vi "fit_fix height and width.vi"() -> ()   [LabVIEW 2016] (continued)
-3.5199999999999996, -3.4799999999999995, -3.4399999999999995, -3.3999999999999995, -3.3600000000000003, -3.3200000000000003, -3.2800000000000002, -3.24, -3.2, -3.16, -3.12, -3.08, -3.04], []}, {[-9.0, -8.96, -8.92, -8.88, -8.84, -8.8, -8.76, -8.72, -8.68, -8.64, -8.6, -8.56, -8.52, -8.48, -8.44, -8.4, -8.36, -8.32, -8.28, -8.24, -8.2, -8.16, -8.12, -8.08, -8.04, -8.0, -7.96, -7.92, -7.88, -7.84, -7.8, -7.76, -7.72, -7.68, -7.64, -7.6, -7.5600000000000005, -7.52, -7.48, -7.4399999999999995, -7.4, -7.359999999999999, -7.32, -7.28, -7.24, -7.2, -7.16, -7.12, -7.08, -7.04, -7.0, -6.96, -6.92, -6.88, -6.84, -6.8, -6.76, -6.72, -6.68, -6.640000000000001, -6.6, -6.5600000000000005, -6.52, -6.48, -6.4399999999999995, -6.4, -6.359999999999999, -6.32, -6.279999999999999, -6.24, -6.199999999999999, -6.16, -6.12, -6.08, -6.04, -6.0, -5.96, -5.92, -5.88, -5.84, -5.8, -5.76, -5.72, -5.68, -5.640000000000001, -5.6, -5.5600000000000005, -5.52, -5.48, -5.4399999999999995, -5.4, -5.359999999999999, -5.32, -5.279999999999999, -5.24, -5.199999999999999, -5.16, -5.12, -5.08, -5.04, -5.0, -4.96, -4.92, -4.88, -4.84, -4.8, -4.76, -4.72, -4.68, -4.64, -4.6, -4.56, -4.52, -4.4799999999999995, -4.4399999999999995, -4.3999999999999995, -4.36, -4.32, -4.28, -4.24, -4.2, -4.16, -4.12, -4.08, -4.04, -4.0, -3.96, -3.92, -3.88, -3.84, -3.8, -3.76, -3.7199999999999998, -3.6799999999999997, -3.6399999999999997, -3.5999999999999996, -3.5599999999999996, -3.5199999999999996, -3.4799999999999995, -3.4399999999999995, -3.3999999999999995, -3.3600000000000003, -3.3200000000000003, -3.2800000000000002, -3.24, -3.2, -3.16, -3.12, -3.08, -3.04], []}, {[-9.0, -8.96, -8.92, -8.88, -8.84, -8.8, -8.76, -8.72, -8.68, -8.64, -8.6, -8.56, -8.52, -8.48, -8.44, -8.4, -8.36, -8.32, -8.28, -8.24, -8.2, -8.16, -8.12, -8.08, -8.04, -8.0, -7.96, -7.92, -7.88, -7.84, -7.8, -7.76, -7.72, -7.68, -7.64, -7.6, -7.5600000000000005, -7.52, -7.48, -7.4399999999999995, -7.4, -7.359999999999999, -7.32, -7.28, -7.24, -7.2, -7.16, -7.12, -7.08, -7.04, -7.0, -6.96, -6.92, -6.88, -6.84, -6.8, -6.76, -6.72, -6.68, -6.640000000000001, -6.6, -6.5600000000000005, -6.52, -6.48, -6.4399999999999995, -6.4, -6.359999999999999, -6.32, -6.279999999999999, -6.24, -6.199999999999999, -6.16, -6.12, -6.08, -6.04, -6.0, -5.96, -5.92, -5.88, -5.84, -5.8, -5.76, -5.72, -5.68, -5.640000000000001, -5.6, -5.5600000000000005, -5.52, -5.48, -5.4399999999999995, -5.4, -5.359999999999999, -5.32, -5.279999999999999, -5.24, -5.199999999999999, -5.16, -5.12, -5.08, -5.04, -5.0, -4.96, -4.92, -4.88, -4.84, -4.8, -4.76, -4.72, -4.68, -4.64, -4.6, -4.56, -4.52, -4.4799999999999995, -4.4399999999999995, -4.3999999999999995, -4.36, -4.32, -4.28, -4.24, -4.2, -4.16, -4.12, -4.08, -4.04, -4.0, -3.96, -3.92, -3.88, -3.84, -3.8, -3.76, -3.7199999999999998, -3.6799999999999997, -3.6399999999999997, -3.5999999999999996, -3.5599999999999996, -3.5199999999999996, -3.4799999999999995, -3.4399999999999995, -3.3999999999999995, -3.3600000000000003, -3.3200000000000003, -3.2800000000000002, -3.24, -3.2, -3.16, -3.12, -3.08, -3.04], []}, {[-9.0, -8.96, -8.92, -8.88, -8.84, -8.8, -8.76, -8.72, -8.68, -8.64, -8.6, -8.56, -8.52, -8.48, -8.44, -8.4, -8.36, -8.32, -8.28, -8.24, -8.2, -8.16, -8.12, -8.08, -8.04, -8.0, -7.96, -7.92, -7.88, -7.84, -7.8, -7.76, -7.72, -7.68, -7.64, -7.6, -7.5600000000000005, -7.52, -7.48, -7.4399999999999995, -7.4, -7.359999999999999, -7.32, -7.28, -7.24, -7.2, -7.16, -7.12, -7.08, -7.04, -7.0, -6.96, -6.92, -6.88, -6.84, -6.8, -6.76, -6.72, -6.68, -6.640000000000001, -6.6, -6.5600000000000005, -6.52, -6.48, -6.4399999999999995, -6.4, -6.359999999999999, -6.32, -6.279999999999999, -6.24, -6.199999999999999, -6.16, -6.12, -6.08, -6.04, -6.0, -5.96, -5.92, -5.88, -5.84, -5.8, -5.76, -5.72, -5.68, -5.640000000000001, -5.6, -5.5600000000000005, -5.52, -5.48, -5.4399999999999995, -5.4, -5.359999999999999, -5.32, -5.279999999999999, -5.24, -5.199999999999999, -5.16, -5.12, -5.08, -5.04, -5.0, -4.96, -4.92, -4.88, -4.84, -4.8, -4.76, -4.72, -4.68, -4.64, -4.6, -4.56, -4.52, -4.4799999999999995, -4.4399999999999995, -4.3999999999999995, -4.36, -4.32, -4.28, -4.24, -4.2, -4.16, -4.12, -4.08, -4.04, -4.0, -3.96, -3.92, -3.88, -3.84, -3.8, -3.76, -3.7199999999999998, -3.6799999999999997, -3.6399999999999997, -3.5999999999999996, -3.5599999999999996, -3.5199999999999996, -3.4799999999999995, -3.4399999999999995, -3.3999999999999995, -3.3600000000000003, -3.3200000000000003, -3.2800000000000002, -3.24, -3.2, -3.16, -3.12, -3.08, -3.04], []}, {[-9.0, -8.96, -8.92, -8.88, -8.84, -8.8, -8.76, -8.72, -8.68, -8.64, -8.6, -8.56, -8.52, -8.48, -8.44, -8.4, -8.36, -8.32, -8.28, -8.24, -8.2, -8.16, -8.12, -8.08, -8.04, -8.0, -7.96, -7.92, -7.88, -7.84, -7.8, -7.76, -7.72, -7.68, -7.64, -7.6, -7.5600000000000005, -7.52, -7.48, -7.4399999999999995, -7.4, -7.359999999999999, -7.32, -7.28, -7.24, -7.2, -7.16, -7.12, -7.08, -7.04, -7.0, -6.96, -6.92, -6.88, -6.84, -6.8, -6.76, -6.72, -6.68, -6.640000000000001, -6.6, -6.5600000000000005, -6.52, -6.48, -6.4399999999999995, -6.4, -6.359999999999999, -6.32, -6.279999999999999, -6.24, -6.199999999999999, -6.16, -6.12, -6.08, -6.04, -6.0, -5.96, -5.92, -5.88, -5.84, -5.8, -5.76, -5.72, -5.68, -5.640000000000001, -5.6, -5.5600000000000005, -5.52, -5.48, -5.4399999999999995, -5.4, -5.359999999999999, -5.32, -5.279999999999999, -5.24, -5.199999999999999, -5.16, -5.12, -5.08, -5.04, -5.0, -4.96, -4.92, -4.88, -4.84, -4.8, -4.76, -4.72, -4.68, -4.64, -4.6, -4.56, -4.52, -4.4799999999999995, -4.4399999999999995, -4.3999999999999995, -4.36, -4.32, -4.28, -4.24, -4.2, -4.16, -4.12, -4.08, -4.04, -4.0, -3.96, -3.92, -3.88, -3.84, -3.8, -3.76, -3.7199999999999998, -3.6799999999999997, -3.6399999999999997, -3.5999999999999996, -3.5599999999999996, -3.5199999999999996, -3.4799999999999995, -3.4399999999999995, -3.3999999999999995, -3.3600000000000003, -3.3200000000000003, -3.2800000000000002, -3.24, -3.2, -3.16, -3.12, -3.08, -3.04], []}, {[-9.0, -8.96, -8.92, -8.88, -8.84, -8.8, -8.76, -8.72, -8.68, -8.64, -8.6, -8.56, -8.52, -8.48, -8.44, -8.4, -8.36, -8.32, -8.28, -8.24, -8.2, -8.16, -8.12, -8.08, -8.04, -8.0, -7.96, -7.92, -7.88, -7.84, -7.8, -7.76, -7.72, -7.68, -7.64, -7.6, -7.5600000000000005, -7.52, -7.48, -7.4399999999999995, -7.4, -7.359999999999999, -7.32, -7.28, -7.24, -7.2, -7.16, -7.12, -7.08, -7.04, -7.0, -6.96, -6.92, -6.88, -6.84, -6.8, -6.76, -6.72, -6.68, -6.640000000000001, -6.6, -6.5600000000000005, -6.52, -6.48, -6.4399999999999995, -6.4, -6.359999999999999, -6.32, -6.279999999999999, -6.24, -6.199999999999999, -6.16, -6.12, -6.08, -6.04, -6.0, -5.96, -5.92, -5.88, -5.84, -5.8, -5.76, -5.72, -5.68, -5.640000000000001, -5.6, -5.5600000000000005, -5.52, -5.48, -5.4399999999999995, -5.4, -5.359999999999999, -5.32, -5.279999999999999, -5.24, -5.199999999999999, -5.16, -5.12, -5.08, -5.04, -5.0, -4.96, -4.92, -4.88, -4.84, -4.8, -4.76, -4.72, -4.68, -4.64, -4.6, -4.56, -4.52, -4.4799999999999995, -4.4399999999999995, -4.3999999999999995, -4.36, -4.32, -4.28, -4.24, -4.2, -4.16, -4.12, -4.08, -4.04, -4.0, -3.96, -3.92, -3.88, -3.84, -3.8, -3.76, -3.7199999999999998, -3.6799999999999997, -3.6399999999999997, -3.5999999999999996, -3.5599999999999996, -3.5199999999999996, -3.4799999999999995, -3.4399999999999995, -3.3999999999999995, -3.3600000000000003, -3.3200000000000003, -3.2800000000000002, -3.24, -3.2, -3.16, -3.12, -3.08, -3.04], []}, {[-9.0, -8.96, -8.92, -8.88, -8.84, -8.8, -8.76, -8.72, -8.68, -8.64, -8.6, -8.56, -8.52, -8.48, -8.44, -8.4, -8.36, -8.32, -8.28, -8.24, -8.2, -8.16, -8.12, -8.08, -8.04, -8.0, -7.96, -7.92, -7.88, -7.84, -7.8, -7.76, -7.72, -7.68, -7.64, -7.6, -7.5600000000000005, -7.52, -7.48, -7.4399999999999995, -7.4, -7.359999999999999, -7.32, -7.28, -7.24, -7.2, -7.16, -7.12, -7.08, -7.04, -7.0, -6.96, -6.92, -6.88, -6.84, -6.8, -6.76, -6.72, -6.68, -6.640000000000001, -6.6, -6.5600000000000005, -6.52, -6.48, -6.4399999999999995, -6.4, -6.359999999999999, -6.32, -6.279999999999999, -6.24, -6.199999999999999, -6.16, -6.12, -6.08, -6.04, -6.0, -5.96, -5.92, -5.88, -5.84, -5.8, -5.76, -5.72, -5.68, -5.640000000000001, -5.6, -5.5600000000000005, -5.52, -5.48, -5.4399999999999995, -5.4, -5.359999999999999, -5.32, -5.279999999999999, -5.24, -5.199999999999999, -5.16, -5.12, -5.08, -5.04, -5.0, -4.96, -4.92, -4.88, -4.84, -4.8, -4.76, -4.72, -4.68, -4.64, -4.6, -4.56, -4.52, -4.4799999999999995, -4.4399999999999995, -4.3999999999999995, -4.36, -4.32, -4.28, -4.24, -4.2, -4.16, -4.12, -4.08, -4.04, -4.0, -3.96, -3.92, -3.88, -3.84, -3.8, -3.76, -3.7199999999999998, -3.6799999999999997, -3.6399999999999997, -3.5999999999999996, -3.5599999999999996, -3.5199999999999996, -3.4799999999999995, -3.4399999999999995, -3.3999999999999995, -3.3600000000000003, -3.3200000000000003, -3.2800000000000002, -3.24, -3.2, -3.16, -3.12, -3.08, -3.04], []}, {[-9.0, -8.96, -8.92, -8.88, -8.84, -8.8, -8.76, -8.72, -8.68, -8.64, -8.6, -8.56, -8.52, -8.48, -8.44, -8.4, -8.36, -8.32, -8.28, -8.24, -8.2, -8.16, -8.12, -8.08, -8.04, -8.0, -7.96, -7.92, -7.88, -7.84, -7.8, -7.76, -7.72, -7.68, -7.64, -7.6, -7.5600000000000005, -7.52, -7.48, -7.4399999999999995, -7.4, -7.359999999999999, -7.32, -7.28, -7.24, -7.2, -7.16, -7.12, -7.08, -7.04, -7.0, -6.96, -6.92, -6.88, -6.84, -6.8, -6.76, -6.72, -6.68, -6.640000000000001, -6.6, -6.5600000000000005, -6.52, -6.48, -6.4399999999999995, -6.4, -6.359999999999999, -6.32, -6.279999999999999, -6.24, -6.199999999999999, -6.16, -6.12, -6.08, -6.04, -6.0, -5.96, -5.92, -5.88, -5.84, -5.8, -5.76, -5.72, -5.68, -5.640000000000001, -5.6, -5.5600000000000005, -5.52, -5.48, -5.4399999999999995, -5.4, -5.359999999999999, -5.32, -5.279999999999999, -5.24, -5.199999999999999, -5.16, -5.12, -5.08, -5.04, -5.0, -4.96, -4.92, -4.88, -4.84, -4.8, -4.76, -4.72, -4.68, -4.64, -4.6, -4.56, -4.52, -4.4799999999999995, -4.4399999999999995, -4.3999999999999995, -4.36, -4.32, -4.28, -4.24, -4.2, -4.16, -4.12, -4.08, -4.04, -4.0, -3.96, -3.92, -3.88, -3.84, -3.8, -3.76, -3.7199999999999998, -3.6799999999999997, -3.6399999999999997, -3.5999999999999996, -3.5599999999999996, -3.5199999999999996, -3.4799999999999995, -3.4399999999999995, -3.3999999999999995, -3.3600000000000003, -3.3200000000000003, -3.2800000000000002, -3.24, -3.2, -3.16, -3.12, -3.08, -3.04], []}, {[-9.0, -8.96, -8.92, -8.88, -8.84, -8.8, -8.76, -8.72, -8.68, -8.64, -8.6, -8.56, -8.52, -8.48, -8.44, -8.4, -8.36, -8.32, -8.28, -8.24, -8.2, -8.16, -8.12, -8.08, -8.04, -8.0, -7.96, -7.92, -7.88, -7.84, -7.8, -7.76, -7.72, -7.68, -7.64, -7.6, -7.5600000000000005, -7.52, -7.48, -7.4399999999999995, -7.4, -7.359999999999999, -7.32, -7.28, -7.24, -7.2, -7.16, -7.12, -7.08, -7.04, -7.0, -6.96, -6.92, -6.88, -6.84, -6.8, -6.76, -6.72, -6.68, -6.640000000000001, -6.6, -6.5600000000000005, -6.52, -6.48, -6.4399999999999995, -6.4, -6.359999999999999, -6.32, -6.279999999999999, -6.24, -6.199999999999999, -6.16, -6.12, -6.08, -6.04, -6.0, -5.96, -5.92, -5.88, -5.84, -5.8, -5.76, -5.72, -5.68, -5.640000000000001, -5.6, -5.5600000000000005, -5.52, -5.48, -5.4399999999999995, -5.4, -5.359999999999999, -5.32, -5.279999999999999, -5.24, -5.199999999999999, -5.16, -5.12, -5.08, -5.04, -5.0, -4.96, -4.92, -4.88, -4.84, -4.8, -4.76, -4.72, -4.68, -4.64, -4.6, -4.56, -4.52, -4.4799999999999995, -4.4399999999999995, -4.3999999999999995, -4.36, -4.32, -4.28, -4.24, -4.2, -4.16, -4.12, -4.08, -4.04, -4.0, -3.96, -3.92, -3.88, -3.84, -3.8, -3.76, -3.7199999999999998, -3.6799999999999997, -3.6399999999999997, -3.5999999999999996, -3.5599999999999996, -3.5199999999999996, -3.4799999999999995, -3.4399999999999995, -3.3999999999999995, -3.3600000000000003, -3.3200000000000003, -3.2800000000000002, -3.24, -3.2, -3.16, -3.12, -3.08, -3.04], []}, {[-9.0, -8.96, -8.92, -8.88, -8.84, -8.8, -8.76, -8.72, -8.68, -8.64, -8.6, -8.56, -8.52, -8.48, -8.44, -8.4, -8.36, -8.32, -8.28, -8.24, -8.2, -8.16, -8.12, -8.08, -8.04, -8.0, -7.96, -7.92, -7.88, -7.84, -7.8, -7.76, -7.72, -7.68, -7.64, -7.6, -7.5600000000000005, -7.52, -7.48, -7.4399999999999995, -7.4, -7.359999999999999, -7.32, -7.28, -7.24, -7.2, -7.16, -7.12, -7.08, -7.04, -7.0, -6.96, -6.92, -6.88, -6.84, -6.8, -6.76, -6.72, -6.68, -6.640000000000001, -6.6, -6.5600000000000005, -6.52, -6.48, -6.4399999999999995, -6.4, -6.359999999999999, -6.32, -6.279999999999999, -6.24, -6.199999999999999, -6.16, -6.12, -6.08, -6.04, -6.0, -5.96, -5.92, -5.88, -5.84, -5.8, -5.76, -5.72, -5.68, -5.640000000000001, -5.6, -5.5600000000000005, -5.52, -5.48, -5.4399999999999995, -5.4, -5.359999999999999, -5.32, -5.279999999999999, -5.24, -5.199999999999999, -5.16, -5.12, -5.08, -5.04, -5.0, -4.96, -4.92, -4.88, -4.84, -4.8, -4.76, -4.72, -4.68, -4.64, -4.6, -4.56, -4.52, -4.4799999999999995, -4.4399999999999995, -4.3999999999999995, -4.36, -4.32, -4.28, -4.24, -4.2, -4.16, -4.12, -4.08, -4.04, -4.0, -3.96, -3.92, -3.88, -3.84, -3.8, -3.76, -3.7199999999999998, -3.6799999999999997, -3.6399999999999997, -3.5999999999999996, -3.5599999999999996, -3.5199999999999996, -3.4799999999999995, -3.4399999999999995, -3.3999999999999995, -3.3600000000000003, -3.3200000000000003, -3.2800000000000002, -3.24, -3.2, -3.16, -3.12, -3.08, -3.04], []}, {[-9.0, -8.96, -8.92, -8.88, -8.84, -8.8, -8.76, -8.72, -8.68, -8.64, -8.6, -8.56, -8.52, -8.48, -8.44, -8.4, -8.36, -8.32, -8.28, -8.24, -8.2, -8.16, -8.12, -8.08, -8.04, -8.0, -7.96, -7.92, -7.88, -7.84, -7.8, -7.76, -7.72, -7.68, -7.64, -7.6, -7.5600000000000005, -7.52, -7.48, -7.4399999999999995, -7.4, -7.359999999999999, -7.32, -7.28, -7.24, -7.2, -7.16, -7.12, -7.08, -7.04, -7.0, -6.96, -6.92, -6.88, -6.84, -6.8, -6.76, -6.72, -6.68, -6.640000000000001, -6.6, -6.5600000000000005, -6.52, -6.48, -6.4399999999999995, -6.4, -6.359999999999999, -6.32, -6.279999999999999, -6.24, -6.199999999999999, -6.16, -6.12, -6.08, -6.04, -6.0, -5.96, -5.92, -5.88, -5.84, -5.8, -5.76, -5.72, -5.68, -5.640000000000001, -5.6, -5.5600000000000005, -5.52, -5.48, -5.4399999999999995, -5.4, -5.359999999999999, -5.32, -5.279999999999999, -5.24, -5.199999999999999, -5.16, -5.12, -5.08, -5.04, -5.0, -4.96, -4.92, -4.88, -4.84, -4.8, -4.76, -4.72, -4.68, -4.64, -4.6, -4.56, -4.52, -4.4799999999999995, -4.4399999999999995, -4.3999999999999995, -4.36, -4.32, -4.28, -4.24, -4.2, -4.16, -4.12, -4.08, -4.04, -4.0, -3.96, -3.92, -3.88, -3.84, -3.8, -3.76, -3.7199999999999998, -3.6799999999999997, -3.6399999999999997, -3.5999999999999996, -3.5599999999999996, -3.5199999999999996, -3.4799999999999995, -3.4399999999999995, -3.3999999999999995, -3.3600000000000003, -3.3200000000000003, -3.2800000000000002, -3.24, -3.2, -3.16, -3.12, -3.08, -3.04], []}, {[-9.0, -8.96, -8.92, -8.88, -8.84, -8.8, -8.76, -8.72, -8.68, -8.64, -8.6, -8.56, -8.52, -8.48, -8.44, -8.4, -8.36, -8.32, -8.28, -8.24, -8.2, -8.16, -8.12, -8.08, -8.04, -8.0, -7.96, -7.92, -7.88, -7.84, -7.8, -7.76, -7.72, -7.68, -7.64, -7.6, -7.5600000000000005, -7.52, -7.48, -7.4399999999999995, -7.4, -7.359999999999999, -7.32, -7.28, -7.24, -7.2, -7.16, -7.12, -7.08, -7.04, -7.0, -6.96, -6.92, -6.88, -6.84, -6.8, -6.76, -6.72, -6.68, -6.640000000000001, -6.6, -6.5600000000000005, -6.52, -6.48, -6.4399999999999995, -6.4, -6.359999999999999, -6.32, -6.279999999999999, -6.24, -6.199999999999999, -6.16, -6.12, -6.08, -6.04, -6.0, -5.96, -5.92, -5.88, -5.84, -5.8, -5.76, -5.72, -5.68, -5.640000000000001, -5.6, -5.5600000000000005, -5.52, -5.48, -5.4399999999999995, -5.4, -5.359999999999999, -5.32, -5.279999999999999, -5.24, -5.199999999999999, -5.16, -5.12, -5.08, -5.04, -5.0, -4.96, -4.92, -4.88, -4.84, -4.8, -4.76, -4.72, -4.68, -4.64, -4.6, -4.56, -4.52, -4.4799999999999995, -4.4399999999999995, -4.3999999999999995, -4.36, -4.32, -4.28, -4.24, -4.2, -4.16, -4.12, -4.08, -4.04, -4.0, -3.96, -3.92, -3.88, -3.84, -3.8, -3.76, -3.7199999999999998, -3.6799999999999997, -3.6399999999999997, -3.5999999999999996, -3.5599999999999996, -3.5199999999999996, -3.4799999999999995, -3.4399999999999995, -3.3999999999999995, -3.3600000000000003, -3.3200000000000003, -3.2800000000000002, -3.24, -3.2, -3.16, -3.12, -3.08, -3.04], []}, {[-9.0, -8.96, -8.92, -8.88, -8.84, -8.8, -8.76, -8.72, -8.68, -8.64, -8.6, -8.56, -8.52, -8.48, -8.44, -8.4, -8.36, -8.32, -8.28, -8.24, -8.2, -8.16, -8.12, -8.08, -8.04, -8.0, -7.96, -7.92, -7.88, -7.84, -7.8, -7.76, -7.72, -7.68, -7.64, -7.6, -7.5600000000000005, -7.52, -7.48, -7.4399999999999995, -7.4, -7.359999999999999, -7.32, -7.28, -7.24, -7.2, -7.16, -7.12, -7.08, -7.04, -7.0, -6.96, -6.92, -6.88, -6.84, -6.8, -6.76, -6.72, -6.68, -6.640000000000001, -6.6, -6.5600000000000005, -6.52, -6.48, -6.4399999999999995, -6.4, -6.359999999999999, -6.32, -6.279999999999999, -6.24, -6.199999999999999, -6.16, -6.12, -6.08, -6.04, -6.0, -5.96, -5.92, -5.88, -5.84, -5.8, -5.76, -5.72, -5.68, -5.640000000000001, -5.6, -5.5600000000000005, -5.52, -5.48, -5.4399999999999995, -5.4, -5.359999999999999, -5.32, -5.279999999999999, -5.24, -5.199999999999999, -5.16, -5.12, -5.08, -5.04, -5.0, -4.96, -4.92, -4.88, -4.84, -4.8, -4.76, -4.72, -4.68, -4.64, -4.6, -4.56, -4.52, -4.4799999999999995, -4.4399999999999995, -4.3999999999999995, -4.36, -4.32, -4.28, -4.24, -4.2, -4.16, -4.12, -4.08, -4.04, -4.0, -3.96, -3.92, -3.88, -3.84, -3.8, -3.76, -3.7199999999999998, -3.6799999999999997, -3.6399999999999997, -3.5999999999999996, -3.5599999999999996, -3.5199999999999996, -3.4799999999999995, -3.4399999999999995, -3.3999999999999995, -3.3600000000000003, -3.3200000000000003, -3.2800000000000002, -3.24, -3.2, -3.16, -3.12, -3.08, -3.04], []}, {[-9.0, -8.96, -8.92, -8.88, -8.84, -8.8, -8.76, -8.72, -8.68, -8.64, -8.6, -8.56, -8.52, -8.48, -8.44, -8.4, -8.36, -8.32, -8.28, -8.24, -8.2, -8.16, -8.12, -8.08, -8.04, -8.0, -7.96, -7.92, -7.88, -7.84, -7.8, -7.76, -7.72, -7.68, -7.64, -7.6, -7.5600000000000005, -7.52, -7.48, -7.4399999999999995, -7.4, -7.359999999999999, -7.32, -7.28, -7.24, -7.2, -7.16, -7.12, -7.08, -7.04, -7.0, -6.96, -6.92, -6.88, -6.84, -6.8, -6.76, -6.72, -6.68, -6.640000000000001, -6.6, -6.5600000000000005, -6.52, -6.48, -6.4399999999999995, -6.4, -6.359999999999999, -6.32, -6.279999999999999, -6.24, -6.199999999999999, -6.16, -6.12, -6.08, -6.04, -6.0, -5.96, -5.92, -5.88, -5.84, -5.8, -5.76, -5.72, -5.68, -5.640000000000001, -5.6, -5.5600000000000005, -5.52, -5.48, -5.4399999999999995, -5.4, -5.359999999999999, -5.32, -5.279999999999999, -5.24, -5.199999999999999, -5.16, -5.12, -5.08, -5.04, -5.0, -4.96, -4.92, -4.88, -4.84, -4.8, -4.76, -4.72, -4.68, -4.64, -4.6, -4.56, -4.52, -4.4799999999999995, -4.4399999999999995, -4.3999999999999995, -4.36, -4.32, -4.28, -4.24, -4.2, -4.16, -4.12, -4.08, -4.04, -4.0, -3.96, -3.92, -3.88, -3.84, -3.8, -3.76, -3.7199999999999998, -3.6799999999999997, -3.6399999999999997, -3.5999999999999996, -3.5599999999999996, -3.5199999999999996, -3.4799999999999995, -3.4399999999999995, -3.3999999999999995, -3.3600000000000003, -3.3200000000000003, -3.2800000000000002, -3.24, -3.2, -3.16, -3.12, -3.08, -3.04], []}]
  out "Initial Parameters":dbl[](array[numeric])=[0.0312226112, 1.0, 0.3242525367447515, 1.0, 0.3675401050825521, 1.0, 0.43936805911250254, 1.0, 0.48162870530723434, 1.0, 0.48518796126797337, 1.0, 0.48518796126797337]
  out "Locations":dbl[](array[numeric])=[0.3242525367447515, 0.33508863417930657, 0.3675401050825521, 0.42821687785510976, 0.43936805911250254, 0.4500743458224035, 0.4660175884542904, 0.48162870530723434, 0.48518796126797337]
  out "Locations index":dbl[](array[numeric])=[16.008910452822743, 22.191667263468158, 40.707517084335, 75.32788962834749, 81.69042395237715, 87.79911460158418, 96.8958574614012, 105.80309917155141, 107.83390538799561]
  in  "STOP":bool
  # "mu: 0.03, 0.02, 0.05\nV: 0.0065, 0.0055, 0.0085"
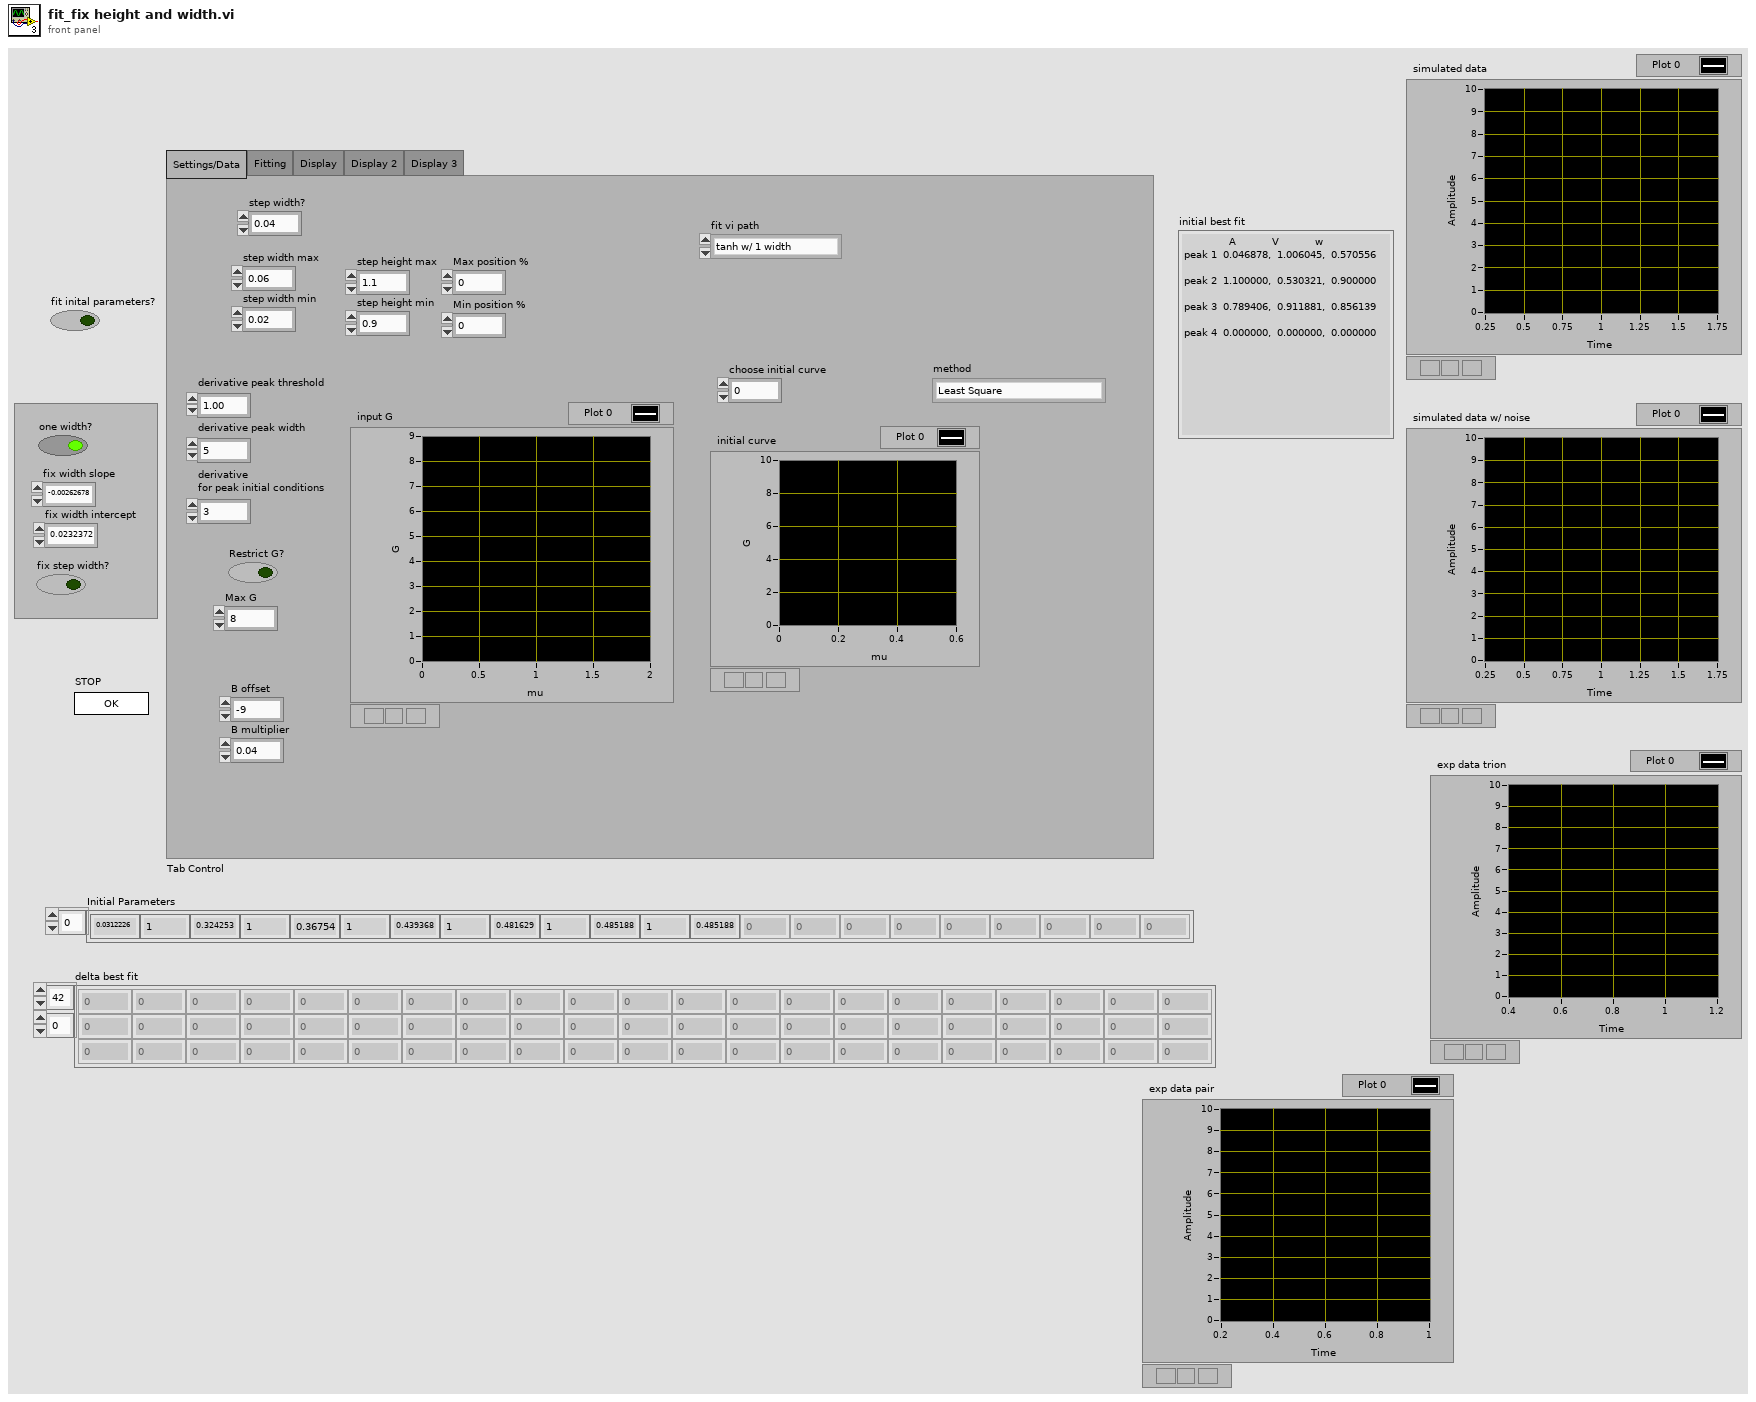
[diagram p1: front panel]
types:
  T1 = enum32{"Settings/Data", "Fitting", "Display", "Display 2", "Display 3"}
  T2 = typedef "NI_AALPro.lvlib/Curve Fitting Criteria.ctl" = u16
  T3 = enum32{"invalid app kind", "Development System", "Run Time System", "Student Edition", "Embedded LabVIEW", "Evaluation", "Custom"}
  T4 = enum32{"Invalid", "Standard", "Closed", "Hidden", "Minimized", "Maximized"}
  T5 = cluster{"Core":cluster{"Current VI Reference":refnum<vi>, "Close Panel on Exit?":bool}, "Done?":bool, "Your string data":string, "All G":cluster{dbl[], dbl[]}[], "Single G curve":cluster{"Single G curve":dbl[], dbl[]}, "Locations index":dbl[], "Locations":dbl[], "Initial Parameters":dbl[], "Best Fit Parameters":dbl[][], "Intermediate Best Fit":dbl[][], "curve #":i32, "fits":cluster{dbl[], dbl[]}[], "intermediate fits":cluster{dbl[], dbl[]}[], "model step #":i32, "parameter bounds":cluster{"parameter minimum":dbl[], "parameter maximum":dbl[]}, "termination":cluster{"max iteration":i32, "tolerance":dbl}, "residues":dbl[], "intermediate residues":dbl[], "fit iteration":i32, "initial curve":cluster{"Single G curve":dbl[], dbl[]}, "Initial curve?":bool, "Initial Best Fit":dbl[], "All locations":dbl[][], "Fit steps":i32[], "one width?":bool, "delta best fit":dbl[][], "Intermediate delta":dbl[][]}
  T6 = cluster{"parameter minimum":dbl[], "parameter maximum":dbl[]}
  T7 = cluster{"Current VI Reference":refnum<vi>, "Close Panel on Exit?":bool}
  T8 = cluster{"Decimated Array":dbl[], "Decimated Array":dbl[]}
  T9 = cluster{"Single G curve":dbl[], "best nonlinear fit":dbl[]}
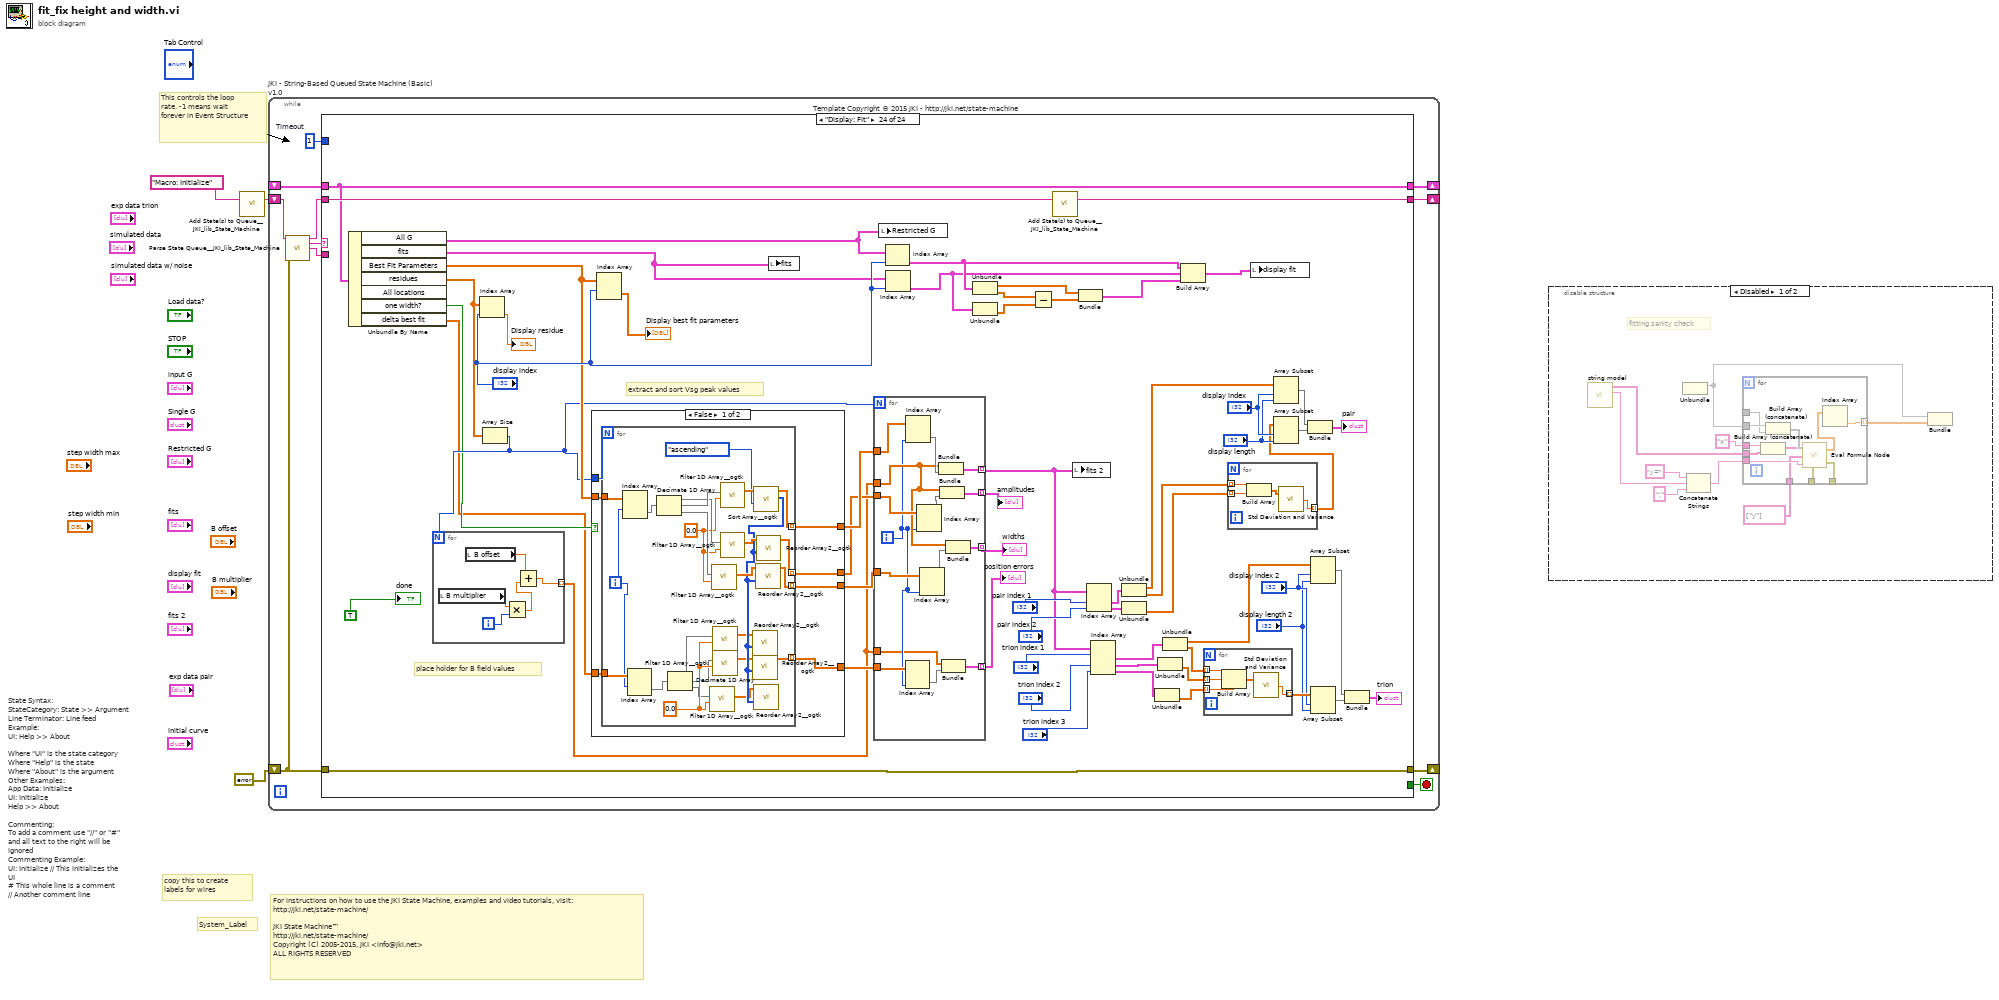
[diagram p0: block diagram]
diagram:
  # "For instructions on how to use the JKI State Machine, examples and video tutorials, visit:\nhttp://jki.net/state-machine/\n\nJKI State Machine™\nhttp://jki.net/state-machine/\nCopyright (C) 2005-2015, JKI <info@jki.net>\nALL RIGHTS RESERVED"
  # "State Syntax:\nStateCategory: State >> Argument\nLine Terminator: Line feed\nExample:\nUI: Help >> About\n\nWhere \"UI\" is the state category\nWhere \"Help\" is the state\nWhere \"About\" is the argument\nOther Examples:\nApp Data: Initialize\nUI: Initialize\nHelp >> About\n\nCommenting:\nTo add a comment use \"//\" or \"#\" and all text to the right will be ignored\nCommenting Example:\nUI: Initialize // This initializes the UI\n# This whole line is a comment\n// Another comment line"
  # "copy this to create labels for wires"
  # "This controls the loop rate. -1 means wait forever in Event Structure"
  # "System_Label"
  n1 = call <vilib>:"Add State(s) to Queue__JKI_lib_State_Machine.vi"("State(s) in (\"\")"="Macro: Initialize") -> ("States Out"=w3:string)  [unwired: 14 in]
  n2 = while "JKI - String-Based Queued State Machine (Basic) v1.0" {
    shift-right: [w7] -> _
    shift-left: _ -> [w6]
    shift-right: [w10] -> _
    shift-left: errorcluster {"status"=FALSE, "code"=0, "source"=""} ("error out") -> [w4]
    shift-right: [w9] -> _
    shift-left: w3 -> [w11]
    stop <- w8 stop-if-true
    w5 = 1  # Timeout
    # "Template Copyright © 2015 JKI - http://jki.net/state-machine"
    n3 = call <vilib>:"Parse State Queue__JKI_lib_State_Machine.vi"("State Queue"=w11, "Error In (no error)"=w4) -> ("Remaining States"=w13:string, "Current State"=w14:string, "Arguments"=w12:string)  [unwired: 11 in]
    n4 = case shown="\"Display: Fit\"" w14 {
      selector: w14 -> [_ _ w66 _ _ _ _ _ _ _ _ _ _ _ _ _ _ _ _ _ _ _ _ _]
      tunnel: w13 -> [w21 w65 w70 w88 w94 w100 w104 w135 w141 w145 w157 w163 w174 w200 w205 w215 w219 w248 w275 w312 w517 w593 w665 w726]
      tunnel: w12 -> [_ _ _ _ _ _ _ _ _ _ _ w158 w168 _ _ _ _ _ _ _ _ _ _ _]
      tunnel: w6 -> [w19 w62 w68 w79 w89 w98 w101 _ w136 w142 w154 w161 w170 w197 w202 w212 w216 w243 w271 w306 w511 w590 w662 w723]
      tunnel: [w18 w63 w72 w85 errorcluster {"status"=FALSE, "code"=0, "source"=""} ("error out") w97 w102 w132 w137 w143 w155 w159 w171 w198 w203 w213 w217 w246 w273 w310 w493 w589 w663 w720] -> w10
      tunnel: w4 -> [w17 w63 w71 w85 w90 w97 w102 w132 w138 w143 w155 w160 w172 w198 w203 w213 w217 w246 w273 w310 w510 w589 w663 w720]
      tunnel: [w20 w64 w69 w87 w93 w99 w103 w134 w140 w144 w156 w162 w173 w199 w204 w214 w218 w247 w274 w311 w516 w592 w664 w725] -> w9
      tunnel: [_ _ _ _ _ TRUE _ _ _ _ _ _ _ _ _ _ _ _ _ _ _ _ _ _] -> w8
      tunnel: [w16 w62 w68 w86 w89 w98 w101 w133 w136 w142 w152 w161 w170 w197 w202 w212 w216 w245 w270 w304 w514 w591 w662 w723] -> w7
      tunnel: w5 -> [w15 _ _ _ _ _ _ _ _ _ _ _ _ _ _ _ _ _ _ _ _ _ _ _]
      frame "", "Event Structure", "Idle" {
        # "executes when the state queue is empty"
        n5 = event shown="[0] Timeout" {
          selector: _ -> [_ _ _ _ _]
          dyn-events: _ -> [_ _ _ _ _]
          timeout: w15 -> [_ _ _ _ _]
          tunnel: w21 -> [w30 w35 w42 w55 w61]
          tunnel: [w29 w34 w41 w54 w60] -> w20
          tunnel: w19 -> [w24 w32 w38 w51 w58]
          tunnel: [w28 w33 w40 w53 w59] -> w18
          tunnel: w17 -> [w28 w33 w40 w53 w59]
          tunnel: [w22 w32 w39 w51 w58] -> w16
          event Timeout {
            n6 = event-data() -> ()  [unwired: 1 in, 1 out]
            n7 = local read "input G"() -> (w26:cluster{dbl[], dbl[]}[])
            n8 = Index Array(array=w26, index="choose initial curve") -> (element=w23:cluster{dbl[], dbl[]})
            n9 = Bundle By Name(cluster=w24, "initial curve"=w23) -> (w22:T5)
            n10 = local write "initial curve"(w23) -> ()
            n11 = call <vilib>:"Add State(s) to Queue__JKI_lib_State_Machine.vi"("State(s) in (\"\")"=w30, "State(s) at Back (\"\")"="Display: Fit" ("State(s) at Back (\"\")")) -> ("States Out"=w29:string)  [unwired: 13 in]
          }
          event "STOP": Value Change {
            # "Exit Button Value Change (pressed) Event\n(this executes Macro: Exit to terminate the VI)"
            n12 = event-data() -> ()  [unwired: 1 in, 1 out]
            n13 = call <vilib>:"Add State(s) to Queue__JKI_lib_State_Machine.vi"("State(s) in Front (\"\")"="Macro: Exit", "State(s) in (\"\")"=w35) -> ("States Out"=w34:string)  [unwired: 13 in]
          }
          event "Load data?": Value Change {
            n14 = event-data() -> ("NewVal"=w36:bool)  [unwired: 1 in, 5 out]
            n15 = case shown="True" w36 {
              tunnel: [w43 w50] -> w39
              tunnel: w38 -> [w43 w49]
              tunnel: [_ "UI: Initialize\nAnalysis: Load data"] -> w37
              frame False {
              }
              frame True {
                w47 = FALSE ("Done?")
                n16 = local write "done"(w47) -> ()
                n17 = Bundle By Name(cluster=w49, "curve #"=0, "Done?"=w47, "fits"=cluster{dbl[], dbl[]}[] [], "Initial curve?"=TRUE) -> (w50:T5)
              }
            }
            n18 = call <vilib>:"Add State(s) to Queue__JKI_lib_State_Machine.vi"("State(s) in Front (\"\")"=w37, "State(s) in (\"\")"=w42) -> ("States Out"=w41:string)  [unwired: 13 in]
          }
          event "display index": Value Change {
            n19 = event-data() -> ()  [unwired: 1 in, 6 out]
            n20 = call <vilib>:"Add State(s) to Queue__JKI_lib_State_Machine.vi"("State(s) in Front (\"\")"="Display: Fit", "State(s) in (\"\")"=w55) -> ("States Out"=w54:string)  [unwired: 13 in]
          }
          event Panel Close? {
            # "Discard the event because we'll close the front panel ourselves in Macro: Exit"
            # "Close Panel button (pressed) Event\n(this executes Macro: Exit to terminate the VI)"
            n21 = event-data() -> ()  [unwired: 1 in, 1 out]
            n22 = event-data("Discard?"=TRUE) -> ()  [unwired: 1 in, 1 out]
            n23 = call <vilib>:"Add State(s) to Queue__JKI_lib_State_Machine.vi"("State(s) in Front (\"\")"="Macro: Exit", "State(s) in (\"\")"=w61) -> ("States Out"=w60:string)  [unwired: 13 in]
          }
        }
      }
      frame "---------- Core ----------" {
        # "Do not put any code in this frame.\n(it is a separator no-op)"
        n24 = call <vilib>:"Add State(s) to Queue__JKI_lib_State_Machine.vi"("State(s) in (\"\")"=w65) -> ("States Out"=w64:string)  [unwired: 14 in]
      }
      frame Default {
        w75 = 42 items=["No error", "Argument error", "Memory is full", "Out of zone", "End of file", "File already open", "Generic file I/O error", "File not found", "File permission error", "Disk is full", "Duplicate path", "Too many files open", "System feature not enabled", "Resource file not found", "Cannot add resource", "Resource not found", "Image not found", "Image memory error", "Pen does not exist", "Config type invalid", "Config token not found", "Config parse error", "Config memory error", "Bad external code format", "Bad external code offset", "External code not present", "Null window", "Destroy window error", "Null menu", "Print aborted", "Bad print record", "Print driver error", "Windows error during printing", "Memory error during printing", "Print dialog error", "Generic print error", "Invalid device refnum", "Device not found", "Device parameter error", "Device unit error", "Cannot open device", "Device call aborted", "Generic error", "Cancelled by user", "Object ID too low", "Object ID too high", "Object not in heap", "Unknown heap", "Unknown object (invalid DefProc)", "Unknown object (DefProc not in table)", "Message out of range", "Invalid (null) method", "Unknown message", "Manager call not supported", "Bad address", "Network operation in progress", "Network operation timed out", "Connection is busy", "Network attribute not supported", "Network error", "Address in use", "System out of memory", "Connection aborted", "Connection refused", "Not connected", "Already connected", "Connection closed", "Initialization error (interapplication manager)", "Bad occurrence", "Wait on unbound occurrence handler", "Occurrence queue overflow", "Datalog type conflict", "Unused", "Unrecognized type (interapplication manager)", "Memory corrupt", "Failed to make temporary DLL", "Old CIN version", "Drag socket not found", "Failed to load drop-object", "Failed to register OLE object", "Failed to release OLE object", "Format specifier type mismatch", "Unknown format specifier", "Too few format specifiers", "Too many format specifiers", "Scan failed", "Newer CIN version", "Error converting to variant", "Runtime menu error", "Password tampered", "Variant attribute not found", "Incompatible variant data type", "Event data is not available", "Event Store is not present", "Occurrence is not found", "Event Queue is not created", "Event info is not available", "Refnum passed is NULL", "Error retrieving Class GUID", "Error retrieving CoClass GUID", "Error retrieving TypeLib GUID.", "Bad built application magic bytes.", "Specific driver is different from the specific driver associated with the Logical Name.", "There is no session opened to the class driver.", "Max Error", "MAX - Error with config objects", "MAX - Error loading configuration", "MAX - Group not supported"]
        # "Current State"
        # "Do not delete, rename, or modify this frame.\n(this is used to capture unhandled states and typos)"
        # "Handle mistyped state name (developer tool)"
        n25 = Format Into String(format string="Software Exception: Unhandled State \"%s\"." ("message"), error in=w71, w66) -> (resulting string=w74:string, error out=w73:errorcluster)  [unwired: 1 in]
        n26 = call <vilib>:"Error Cluster From Error Code.vi"("show call chain? (False)"=TRUE, "error in (no error)"=w73, "error message (\"\")"=w74, "error code (0)"=w75) -> ("error out"=w72:errorcluster)  [unwired: 5 in]
        n27 = call <vilib>:"Add State(s) to Queue__JKI_lib_State_Machine.vi"("State(s) in (\"\")"=w70) -> ("States Out"=w69:string)  [unwired: 14 in]
      }
      frame "Initialize Core Data" {
        # "Do not delete, rename, or modify this frame.\n(this is used to determine panel behavior on exit)"
        # "originally closed?"
        # "exe?"
        # "If panel starts closed or is an EXE, then close it when we exit"
        n28 = property class="VI"() -> ("Front Panel.Open"=w84:bool)  [unwired: 2 in, 2 out]
        n29 = property class="App"() -> ("App.Kind"=w83:T3)  [unwired: 2 in, 2 out]
        n30 = control-ref of="Current VI Reference"() -> (w77:refnum<vi>)
        n31 = Not(x=w84) -> (.not. x?=w81:bool)
        n32 = Equal?(x=w83, y=T3."Run Time System" ("Application:Kind")) -> (x = y?=w80:bool)
        n33 = Or(x=w81, y=w80) -> (x .or. y?=w78:bool)
        n34 = Bundle By Name(cluster=w79, "Core.Current VI Reference"=w77, "Core.Close Panel on Exit?"=w78) -> (w86:T5)
        n35 = call <vilib>:"Add State(s) to Queue__JKI_lib_State_Machine.vi"("State(s) in (\"\")"=w88) -> ("States Out"=w87:string)  [unwired: 14 in]
      }
      frame "Error Handler" {
        # "Unhandled Error -- Display it"
        # "Handle any errors here.\nYou can also output any states to clean-up after errors occur"
        # "Clear error"
        n36 = disable-structure shown="Disabled" {
          disable-tunnel: w90 -> [w95 _]
          frame Disabled {
            n37 = call <vilib>:"General Error Handler.vi"("error in (no error)"=w95) -> ()  [unwired: 10 in, 5 out]
          }
          frame Enabled {
          }
        }
        n38 = call <vilib>:"Add State(s) to Queue__JKI_lib_State_Machine.vi"("State(s) in (\"\")"=w94, "State(s) at Back (\"\")"="/* Post Error States") -> ("States Out"=w93:string)  [unwired: 13 in]
      }
      frame "Exit" {
        # "Do not put any code in this frame.\n(No errors that occur here will be handled.)"
        n39 = call <vilib>:"Add State(s) to Queue__JKI_lib_State_Machine.vi"("State(s) in (\"\")"=w100) -> ("States Out"=w99:string)  [unwired: 14 in]
      }
      frame "---------- Data ----------" {
        # "Do not put any code in this frame.\n(It is a separator no-op. You can make a copy of this frame to create a new Data frame)"
        n40 = call <vilib>:"Add State(s) to Queue__JKI_lib_State_Machine.vi"("State(s) in (\"\")"=w104) -> ("States Out"=w103:string)  [unwired: 14 in]
      }
      frame "Data: Initialize" {
        w105 = dbl[][] []  # delta best fit
        w106 = dbl[][] []  # Intermediate delta
        w107 = FALSE  # one width?
        w108 = i32[] []  # Fit steps
        w109 = dbl[][] []  # All locations
        w110 = dbl[] []  # Initial Best Fit
        w111 = FALSE  # Initial curve?
        w112 = cluster{"Single G curve":dbl[], dbl[]} {"Single G curve"=[], []}  # initial curve
        w114 = dbl[] []  # intermediate residues
        w115 = cluster{dbl[], dbl[]}[] []  # intermediate fits
        w116 = dbl[][] []  # Intermediate Best Fit
        w118 = 0  # fit iteration
        w119 = dbl[] []  # residues
        w120 = cluster{"max iteration":i32, "tolerance":dbl} {"max iteration"=200, "tolerance"=1e-08}  # termination
        w121 = T6 {"parameter minimum"=[], "parameter maximum"=[]}  # parameter bounds
        w122 = 0  # model step #
        w123 = dbl[][] []  # Best Fit Parameters
        w124 = dbl[] []  # Initial Parameters
        w125 = dbl[] []  # Locations
        w126 = dbl[] []  # Locations index
        w117 = -1  # curve #
        w127 = cluster{"Single G curve":dbl[], dbl[]} {"Single G curve"=[], []}  # Single G curve
        w128 = cluster{dbl[], dbl[]}[] []  # All G
        w129 = T7 {"Current VI Reference"=refnum, "Close Panel on Exit?"=FALSE}  # Core
        w131 = TRUE  # Done?
        w130 = ""  # Your string data
        # "Initialize the shift-register data, here.\n(data names are defined by what you wire into the bundle function)"
        n41 = local read "fits"() -> (w113:cluster{dbl[], dbl[]}[])
        n42 = call <vilib>:"Add State(s) to Queue__JKI_lib_State_Machine.vi"("State(s) in (\"\")"=w135) -> ("States Out"=w134:string)  [unwired: 14 in]
        n43 = Bundle("Core"=w129, "Done?"=w131, "Your string data"=w130, "All G"=w128, "Single G curve"=w127, "Locations index"=w126, "Locations"=w125, "Initial Parameters"=w124, "Best Fit Parameters"=w123, "Intermediate Best Fit"=w116, "curve #"=w117, "fits"=w113, "intermediate fits"=w115, "model step #"=w122, "parameter bounds"=w121, "termination"=w120, "residues"=w119, "intermediate residues"=w114, "fit iteration"=w118, "initial curve"=w112, "Initial curve?"=w111, "Initial Best Fit"=w110, "All locations"=w109, "Fit steps"=w108, "one width?"=w107, "delta best fit"=w105, "Intermediate delta"=w106) -> (w133:T5)  [unwired: 1 in]
      }
      frame "Data: Cleanup" {
        # "Cleanup any data and references, here.\n(this is called automatically, by the Macro: Exit)"
        n44 = Unbundle By Name(w136) -> ("Core.Current VI Reference"=w139:refnum<vi>)
        n45 = Close Reference(reference=w139, error in (no error)=w138) -> (error out=w137:errorcluster)
        n46 = call <vilib>:"Add State(s) to Queue__JKI_lib_State_Machine.vi"("State(s) in (\"\")"=w141) -> ("States Out"=w140:string)  [unwired: 14 in]
      }
      frame "---------- UI ----------" {
        # "Do not put any code in this frame.\n(It is a separator no-op. You can make a copy of this frame to create a new UI frame)"
        n47 = call <vilib>:"Add State(s) to Queue__JKI_lib_State_Machine.vi"("State(s) in (\"\")"=w145) -> ("States Out"=w144:string)  [unwired: 14 in]
      }
      frame "UI: Initialize" {
        # "default termination conditions"
        # "Initialize the User Interface, here.\n(this is called automatically, by the Macro: Init)"
        n48 = Bundle By Name(cluster=w154, "intermediate fits"=cluster{dbl[], dbl[]}[] [] ("fits"), "Best Fit Parameters"=dbl[][] [], "Intermediate Best Fit"=dbl[][] [] ("Best Fit Parameters"), "residues"=dbl[] [], "fit iteration"=0, "termination"=cluster{"max iteration":i32, "tolerance":dbl} {"max iteration"=200, "tolerance"=1e-08}, "Fit steps"=i32[] []) -> (w152:T5)
        n49 = call <vilib>:"Add State(s) to Queue__JKI_lib_State_Machine.vi"("State(s) in (\"\")"=w157) -> ("States Out"=w156:string)  [unwired: 14 in]
      }
      frame "UI: Cursor Set" {
        # "Argument"
        # "Set and Unset Cursor Busy.\n(Usage: \"UI: Cursor Set >> Busy|Idle\")"
        n50 = case shown="\"Idle\", Default" w158 {
          tunnel: w160 -> [w165 w167]
          tunnel: [w164 w166] -> w159
          frame "Idle", Default {
            n51 = call <vilib>:"Unset Busy.vi"("error in (no error)"=w165) -> ("error out"=w164:errorcluster)  [unwired: 10 in]
          }
          frame "Busy" {
            n52 = call <vilib>:"Set Busy.vi"("error in (no error)"=w167) -> ("error out"=w166:errorcluster)  [unwired: 9 in, 1 out]
          }
        }
        n53 = call <vilib>:"Add State(s) to Queue__JKI_lib_State_Machine.vi"("State(s) in (\"\")"=w163) -> ("States Out"=w162:string)  [unwired: 14 in]
      }
      frame "UI: Front Panel State" {
        # "Argument"
        # "Set Front Panel Open or Closed\n(Usage: \"UI: Front Panel State >> Open|Close\")"
        n54 = Unbundle By Name(w170) -> ("Core.Current VI Reference"=w169:refnum<vi>)
        n55 = case shown="\"Open\", Default" w168 {
          tunnel: w172 -> [w178 w191]
          tunnel: [w180 w192] -> w171
          tunnel: w169 -> [w179 w189]
          frame "Open", Default {
            n56 = property class="VI"(reference=w179, error in=w178) -> (reference out=w176:refnum<vi>, error out=w177:errorcluster, "Front Panel.Open"=w175:bool)
            n57 = case shown="False" w175 {
              tunnel: [w183 w186] -> w180
              tunnel: w177 -> [w182 w186]
              tunnel: w176 -> [w181 _]
              frame False {
                n58 = invoke class="VI" method="FP.Open"(reference=w181, error in=w182, "Activate"=TRUE, "State"=T4."Standard") -> (error out=w183:errorcluster)  [unwired: 1 in, 4 out]
              }
              frame True {
              }
            }
          }
          frame "Close" {
            n59 = property class="VI"(reference=w189, error in=w191) -> (reference out=w188:refnum<vi>, error out=w190:errorcluster, "Front Panel.Open"=w187:bool)
            n60 = case shown="True" w187 {
              tunnel: [w193 w196] -> w192
              tunnel: w190 -> [w193 w195]
              tunnel: w188 -> [_ w194]
              frame False {
              }
              frame True {
                n61 = invoke class="VI" method="FP.Close"(reference=w194, error in=w195) -> (error out=w196:errorcluster)  [unwired: 1 in, 2 out]
              }
            }
          }
        }
        n62 = call <vilib>:"Add State(s) to Queue__JKI_lib_State_Machine.vi"("State(s) in (\"\")"=w174) -> ("States Out"=w173:string)  [unwired: 14 in]
      }
      frame "---------- Macro ----------" {
        # "Do not put any code in this frame.\n(It is a separator no-op. You can make a copy of this frame to create a new Macro frame)"
        n63 = call <vilib>:"Add State(s) to Queue__JKI_lib_State_Machine.vi"("State(s) in (\"\")"=w200) -> ("States Out"=w199:string)  [unwired: 14 in]
      }
      frame "Macro: Initialize" {
        w201 = "Data: Initialize\nInitialize Core Data\nUI: Initialize\nUI: Front Panel State >> Open"  # Data: Initialize Initialize Core Data UI: Initialize UI: Front Panel State >> Open
        # "Initialization Macro\n(This is called once, when the VI starts)"
        n64 = call <vilib>:"Add State(s) to Queue__JKI_lib_State_Machine.vi"("State(s) in Front (\"\")"=w201, "State(s) in (\"\")"=w205) -> ("States Out"=w204:string)  [unwired: 13 in]
      }
      frame "Macro: Exit" {
        # "Exit Macro\n(This is called once, when the VI exits)"
        n65 = Unbundle By Name(w212) -> ("Core.Close Panel on Exit?"=w211:bool)
        n66 = Select(t="UI: Front Panel State >> Close", s=w211, f="") -> (s? t:f=w208:string)
        n67 = call <vilib>:"Add State(s) to Queue__JKI_lib_State_Machine.vi"("State(s) in (\"\")"=w208, "State(s) at Back (\"\")"="Data: Cleanup\nExit") -> ("States Out"=w206:string)  [unwired: 13 in]
